vi "is a 2D-array.vi"(1 "Values":dbl[][](array[numeric])) -> (0 "2D-Array?":bool)   [LabVIEW 2019]
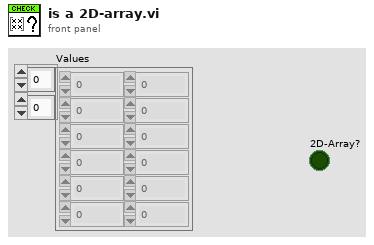
[diagram p1: front panel]
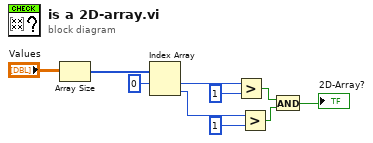
[diagram p0: block diagram]
diagram:
  n1 = Array Size(array="Values") -> (size(s)=w9:i32[])
  n2 = Index Array(array=w9, index #1=0 ("index")) -> (element #1=w7:i32, element #2=w4:i32)  [unwired: 1 in]
  n3 = Greater?(x=w7, y=1) -> (0:w2:bool)
  n4 = Greater?(x=w4, y=1) -> (0:w3:bool)
  n5 = And(x=w2, y=w3) -> (x .and. y?=→"2D-Array?":bool)
